vi "Disabled.vi"(7 "Robot Mode":T2, 10 "Match Info":T1={"Autonomous Elapsed Seconds"=0.0, "TeleOp Elapsed Seconds"=0.0, "Disabled Elapsed Seconds"=0.0, "Visited Autonomous"=FALSE, "Visited TeleOp"=FALSE, "Visited Disabled"=FALSE, "Autonomous Settings"={"Autonomous Style"=enum."Independent", "VI Refnum"=refnum}}, 11 "Call Context":T3) -> ()   [LabVIEW 2018]
doc: "This VI is called each time a disabled packet is received from the DS. It can be used to prepare for the next robot mode, to calibrate sensors, etc."
uses:
  <vilib>/Rock Robotics/WPI/DriverStation/WPI_DriverStationDerivedRobotMode.ctl
  <vilib>/Rock Robotics/WPI/DriverStation/WPI_DriverStationRobotMode2.ctl
  <vilib>/Rock Robotics/WPI/DriverStation/WPI_DriverStationMatch Info.ctl
  <vilib>/Rock Robotics/Network Tables/NT Read Number.vi
  Robot Global Data.vi
  <vilib>/Rock Robotics/Network Tables/NT Write Number.vi
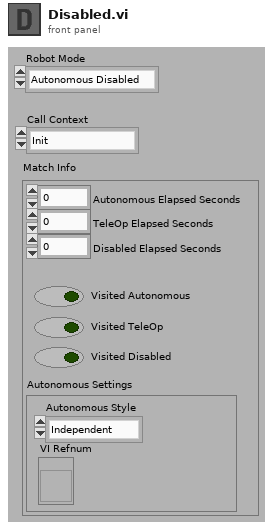
[diagram p1: front panel]
types:
  T1 = typedef "WPI_DriverStationMatch Info.ctl" = cluster{"Autonomous Elapsed Seconds":dbl, "TeleOp Elapsed Seconds":dbl, "Disabled Elapsed Seconds":dbl, "Visited Autonomous":bool, "Visited TeleOp":bool, "Visited Disabled":bool, "Autonomous Settings":cluster{"Autonomous Style":enum16{"Iterative", "Independent"}, "VI Refnum":refnum<vi>}}
  T2 = typedef "WPI_DriverStationRobotMode2.ctl" = enum16{"Autonomous Disabled", "Autonomous Enabled", "Teleop Disabled", "Teleop Enabled", "Disconnected", "Finish", "Test Disabled", "Test Enabled", "Emergency Stopped"}
  T3 = typedef "WPI_DriverStationDerivedRobotMode.ctl" = enum16{"Init", "Execute", "Stop"}
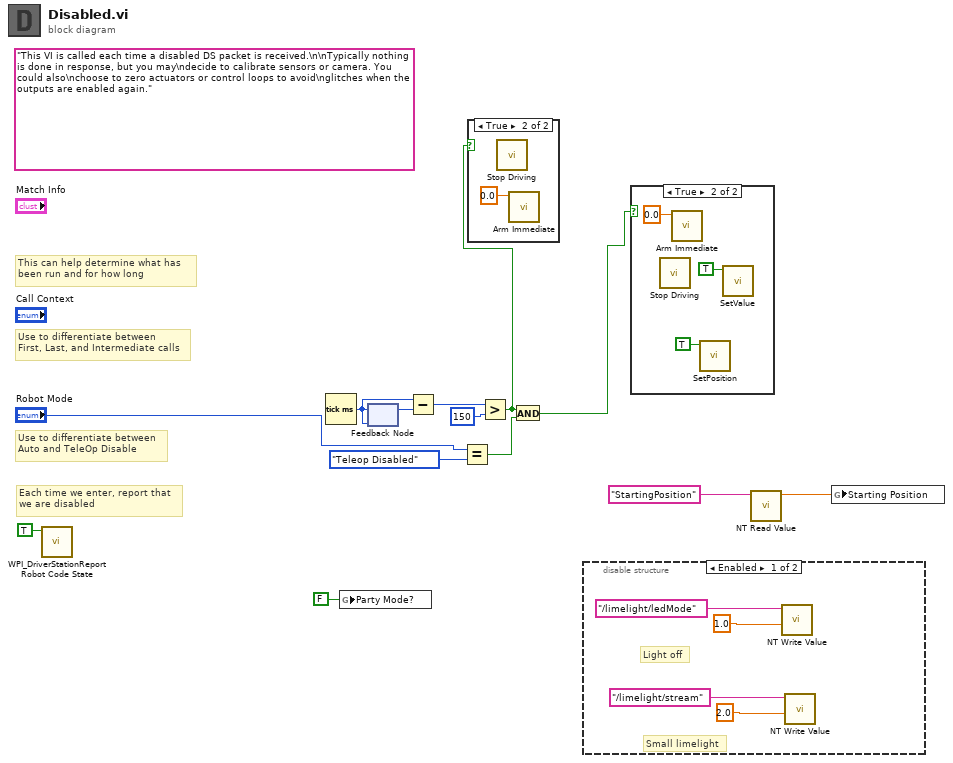
[diagram p0: block diagram]
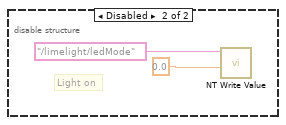
[diagram p3: hidden frame]
diagram:
  (unwired) "This VI is called each time a disabled DS packet is received.\n\nTypically nothing is done in response, but you may\ndecide to calibrate sensors or camera. You could also\nchoose to zero actuators or control loops to avoid\nglitches when the outputs are enabled again."
  # "Each time we enter, report that\nwe are disabled"
  # "Use to differentiate between\nFirst, Last, and Intermediate calls"
  # "This can help determine what has\nbeen run and for how long"
  # "Use to differentiate between\nAuto and TeleOp Disable"
  n1 = call <vilib>:"WPI_DriverStationReport Robot Code State.vi"("Disabled"=TRUE ("Autonomous")) -> ()  [unwired: 10 in, 1 out]
  n2 = Tick Count (ms)() -> (millisecond timer value=w11:u32)
  n3 = global write "Robot Global Data.vi" "Party Mode?"(FALSE) -> ()
  n4 = feedback-in #1(w11) -> ()
  n5 = feedback #1(w11) -> (w12:u32)
  n6 = Subtract(x=w11, y=w12) -> (x-y=w8:u32)
  n7 = Equal?(x="Robot Mode", y=WPI_DriverStationRobotMode2."Teleop Disabled") -> (x = y?=w10:bool)
  n8 = Greater?(x=w8, y=u32 150) -> (0:w2:bool)
  n9 = case shown="True" w2 {
    frame False {
    }
    frame True {
      n10 = call "Stop Driving.vi"() -> ()  [unwired: 11 in, 1 out]
      n11 = call "Arm Immediate.vi"("Speed"=0.0) -> ()  [unwired: 10 in, 1 out]
    }
  }
  n12 = And(x=w2, y=w10) -> (x .and. y?=w6:bool)
  n13 = disable-structure shown="Enabled" {
    frame Enabled {
      # "Small limelight"
      # "Light off"
      n14 = call-poly <vilib>:"NT Write Value.vi"("Numeric"=1.0, "Name"="/limelight/ledMode") -> ()  [unwired: 9 in, 1 out]
      n15 = call-poly <vilib>:"NT Write Value.vi"("Numeric"=2.0, "Name"="/limelight/stream") -> ()  [unwired: 9 in, 1 out]
    }
    frame Disabled {
      # "Light on"
      n16 = call-poly <vilib>:"NT Write Value.vi"("Numeric"=0.0, "Name"="/limelight/ledMode") -> ()  [unwired: 9 in, 1 out]
    }
  }
  n17 = case shown="True" w6 {
    frame False {
    }
    frame True {
      n18 = call "Stop Driving.vi"() -> ()  [unwired: 11 in, 1 out]
      n19 = call "Arm Immediate.vi"("Speed"=0.0) -> ()  [unwired: 10 in, 1 out]
      n20 = call "SetPosition.vi"("Down and out?"=TRUE) -> ()  [unwired: 10 in, 1 out]
      n21 = call "SetValue.vi"("Value"=TRUE) -> ()  [unwired: 10 in, 1 out]
    }
  }
  n22 = call-poly <vilib>:"NT Read Value.vi"("Name"="StartingPosition") -> ("Numeric"=w4:dbl)  [unwired: 9 in, 1 out]
  n23 = global write "Robot Global Data.vi" "Starting Position"(w4) -> ()
